vi "AutotoolRegions.vi"(5 "XRef":refnum<vi>, 6 "State In":T1={"Input Type"=variant(dbl 0.0), "Selection"=0, "Element Names"=[], "Type Strings"=[], "Element Types"=[]}) -> (2 "Regions":T2)   [LabVIEW 2015, in "Construct-Tagged-Union.xnode"]
doc: "This ability VI is called by LabVIEW to determine which tool to use when hovering over an xnode in edit mode, if autotool is turned on. The Bounds of each region is a rectangular region of the xnode in coordinates relative to the top left corner of the xnode. Tool is the autotool that should be used when the user hovers over the particular region of the xnode.\n \n LabVIEW will sort the Regions by Priority so that lower priority regions are tried first in determining what tool to use.\n \n This VI cannot override autotool behavior on grow handles and terminal whiskers of xnodes.\n \n LabVIEW may cache the Regions array and can also call this VI if the Regions array is not currently cached. To force LabVIEW to call this VI and update its autotool regions, use the Reply of \"UpdateAutotoolRegions\".\n\nDefault behavior: None.\n\nThis ability does not provide UI and OS messages are not handled."
uses:
  Construct-Tagged-Union.xnode
  <vilib>/XNodeSupport/XNodeAutotoolRegions.ctl
  <vilib>/XNodeSupport/XNodeAutotoolRegion.ctl
  <vilib>/XNodeSupport/XNodeRect32.ctl
  <vilib>/XNodeSupport/XNodeInt.ctl
  <vilib>/XNodeSupport/XNodeTools.ctl
  State.ctl
  <vilib>/XNodeSupport/NI_XNodeSupport.lvlib
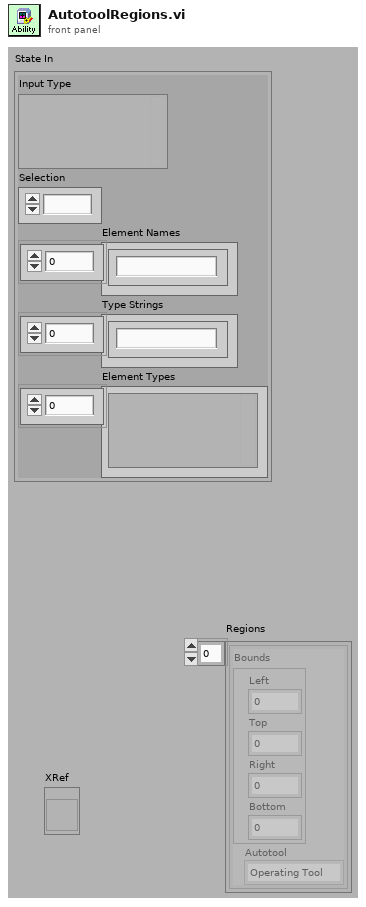
[diagram p1: front panel]
types:
  T1 = typedef "Construct-Tagged-Union.xnode/State.ctl" = cluster{"Input Type":variant, "Selection":i32, "Element Names":string[], "Type Strings":string[], "Element Types":variant[]}
  T2 = typedef "NI_XNodeSupport.lvlib/XNodeAutotoolRegions.ctl" = T3[]
  T3 = typedef "NI_XNodeSupport.lvlib/XNodeAutotoolRegion.ctl" = cluster{"Bounds":T4, "Autotool":T6}
  T4 = typedef "NI_XNodeSupport.lvlib/XNodeRect32.ctl" = cluster{"Left":T5, "Top":T5, "Right":T5, "Bottom":T5}
  T5 = typedef "NI_XNodeSupport.lvlib/XNodeInt.ctl" = i32
  T6 = typedef "NI_XNodeSupport.lvlib/XNodeTools.ctl" = enum32{"Operating Tool", "Placement Tool", "Labelling Tool", "Wiring Tool", "Scroll Tool", "Breakpoint Tool", "Probe Tool", "Auto Tool"}
  T7 = cluster{"left":i16, "top":i16, "right":i16, "bottom":i16}
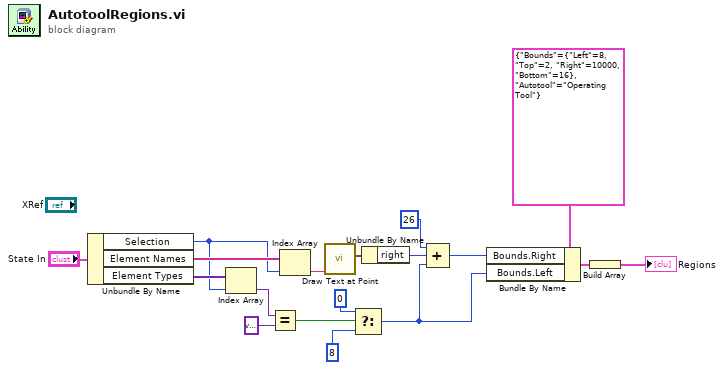
[diagram p0: block diagram]
diagram:
  n1 = Unbundle By Name("State In") -> ("Selection"=w10:i32, "Element Names"=w15:string[], "Element Types"=w11:variant[])
  n2 = Index Array(array=w11, index=w10) -> (element=w9:variant)
  n3 = Equal?(x=w9, y=variant) -> (x = y?=w7:bool)
  n4 = Index Array(array=w15, index=w10) -> (element=w14:string)
  n5 = call <vilib>:"Draw Text at Point.vi"("text"=w14) -> ("text rect"=w13:T7)  [unwired: 9 in, 1 out]
  n6 = Select(t=i16 0 ("x"), s=w7, f=i16 8 ("x")) -> (s? t:f=w3:i16)
  n7 = Unbundle By Name(w13) -> ("right"=w12:i16)
  n8 = Compound Arithmetic op=ADD(i16 26 ("value"), w12, w3) -> (w1:i16)
  n9 = Bundle By Name(cluster=T3 {"Bounds"={"Left"=8, "Top"=2, "Right"=10000, "Bottom"=16}, "Autotool"=enum."Operating Tool"} ("Autotool Region"), "Bounds.Right"=w1, "Bounds.Left"=w3) -> (w17:T3)
  n10 = Build Array(w17) -> (→"Regions":T3[])
